vi "Binary_SpectroscopyFile-ExportSlices.vi"() -> ()   [LabVIEW 2016]
doc: "Opens a binary spectroscopy file, then it loops over all spectroscopy experiments doing the following:\n\n - read spectroscopy data\n - extract slices at the specified Sweep signal values in Slices @ control\n - export slices as a scan data file (.sxm, like the files created by the Scan control module) or in\n ASCII format (with a header and several tab-separated data columns)\n\n- Nanonis Programming Interface -"
uses:
  Nanonis Prog Interface.lvlib
  <vilib>/Analysis/NI_AALPro.lvlib
panel:
  in  "Clear Slices array":bool
  in  "Fill Slices array":bool
  out "Points":i32
  out "Sweep signal":string
  out "Sweep End":sgl format="%.2p"
  out "Sweep Start":sgl format="%.2p"
  in  "Export as":enum16{"sxm (scan file)", "ASCII"}(ring)
  out "Status":string
  in  "Filter":bool
  in  "Slices @":dbl[](array[numeric]) caption="m" format="%#_5p"
  in  "Stop":bool
  in  "Channel":u16(ring) items=["Current (A)", "Current [bwd] (A)"]
  in  "Save":bool
  in  "Filter configuration":T1={"Window width\n(# Points for fit)"=20, "Polynomial order"=3}
  out "Error out":errorcluster
  in  "Binary Spectroscopy file path":path
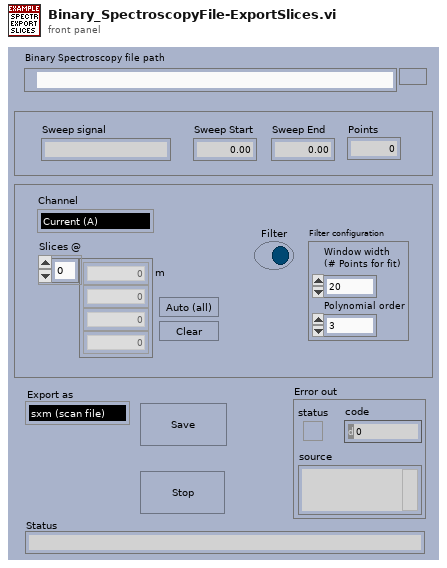
[diagram p1: front panel]
types:
  T1 = cluster{"Window width\n(# Points for fit)":i32, "Polynomial order":i32}
  T2 = enum16{"open", "open or create", "create or replace", "create", "open (read only)"}
  T3 = enum32{"SVD", "Givens", "Givens2", "Householder", "LU Decomposition", "Cholesky"}
  T4 = typedef "Nanonis Prog Interface.lvlib/Binary_SpectroscopyFile-Config.ctl" = cluster{"Num Par":i32, "Exp size":i32, "Points":i32, "Grid Dim X":i32, "Grid Dim Y":i32, "Header size":i32, "Channels":string[], "Parameters":string[], "Sweep Signal":string, "Grid":cluster{"center X (m)":sgl, "center Y (m)":sgl, "width (m)":sgl, "height (m)":sgl, "angle (deg)":sgl}}
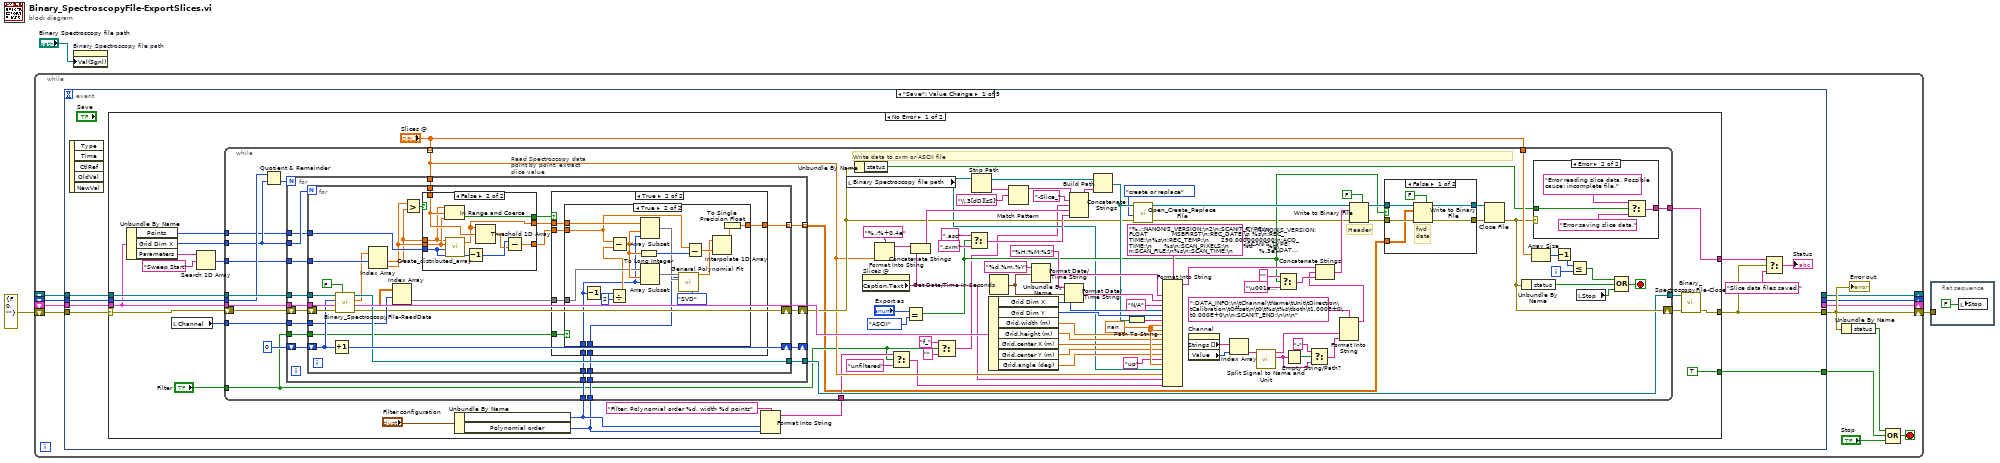
[diagram p0: block diagram]
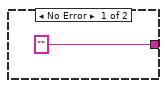
[diagram p2: hidden frame]
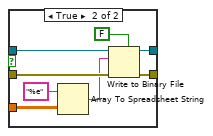
[diagram p3: hidden frame]
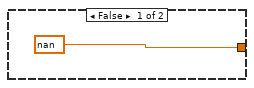
[diagram p4: hidden frame]
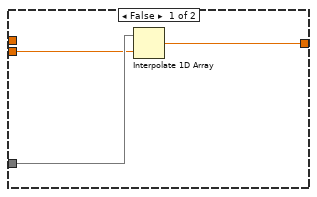
[diagram p5: hidden frame]
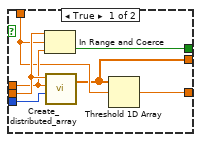
[diagram p6: hidden frame]
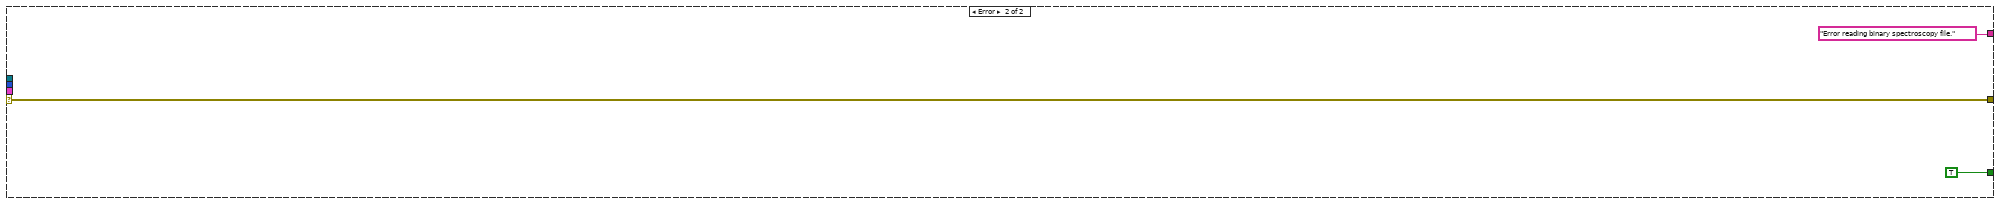
[diagram p7: hidden frame]
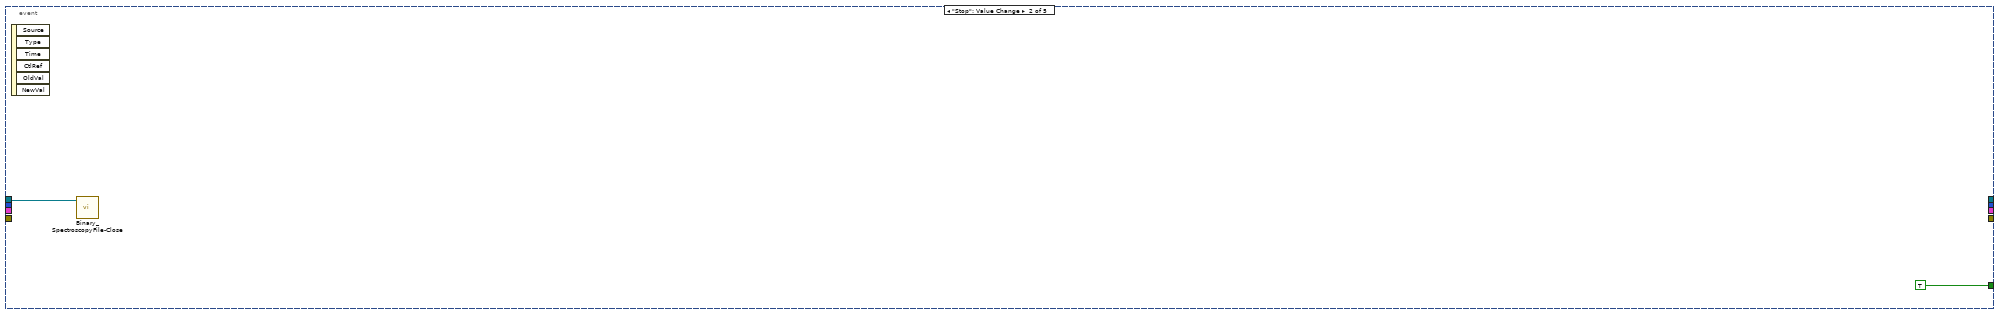
[diagram p8: hidden frame]
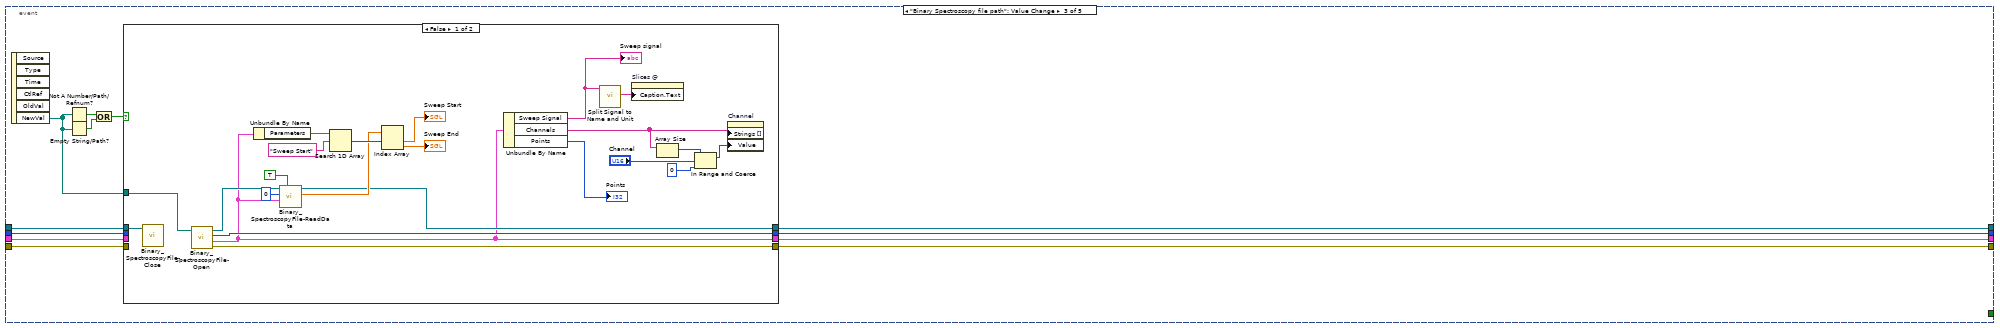
[diagram p9: hidden frame]
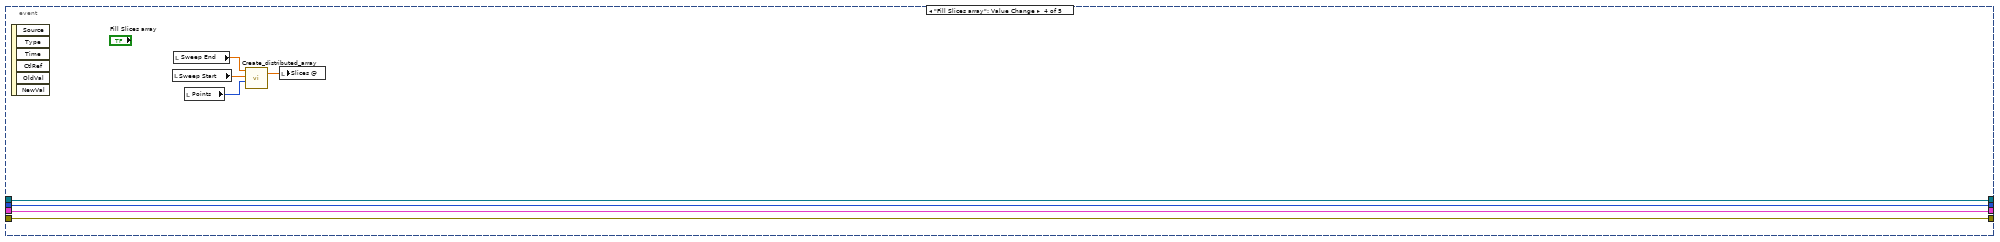
[diagram p11: hidden frame]
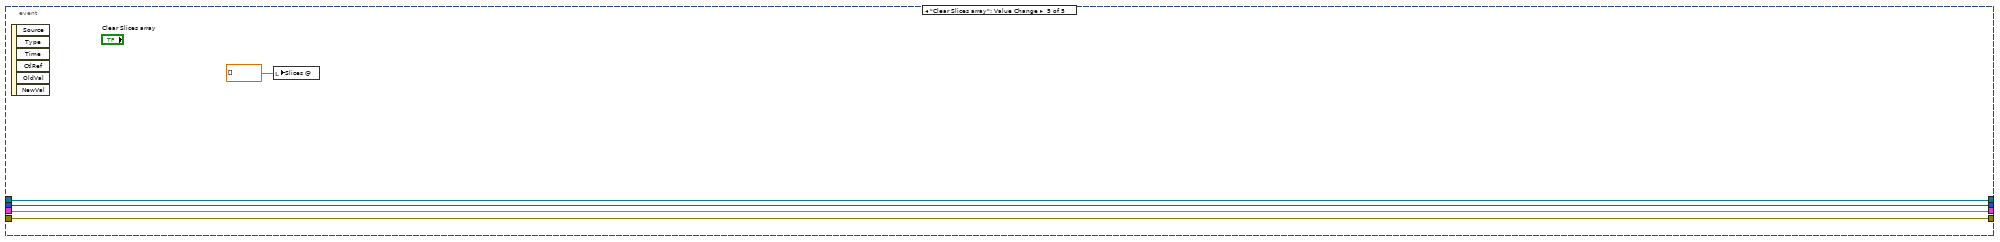
[diagram p12: hidden frame]
diagram:
  n1 = while {
    shift-right: [w4] -> _
    shift-left: _ -> [w8]
    shift-right: [w5] -> _
    shift-left: _ -> [w9]
    shift-right: [w6] -> _
    shift-left: _ -> [w10]
    shift-right: [w7] -> w3
    shift-left: errorcluster {"status"=FALSE, "code"=0, "source"=""} ("error out") -> [w11]
    stop <- w15 stop-if-true
    n2 = event shown="[0] \"Save\": Value Change" {
      selector: _ -> [_ _ _ _ _]
      dyn-events: _ -> [_ _ _ _ _]
      timeout: _ -> [_ _ _ _ _]
      tunnel: [w24 TRUE _ _ _] -> w12
      tunnel: w11 -> [w23 _ w248 w291 w296]
      tunnel: w10 -> [w22 _ w249 w292 w297]
      tunnel: w9 -> [w21 _ w250 w293 w298]
      tunnel: w8 -> [w20 w246 w251 w294 w299]
      tunnel: [w19 _ w256 w291 w296] -> w7
      tunnel: [_ _ w257 w292 w297] -> w6
      tunnel: [_ _ w258 w293 w298] -> w5
      tunnel: [_ _ w259 w294 w299] -> w4
      event "Save": Value Change {
        n3 = event-data() -> ()  [unwired: 1 in, 5 out]
        n4 = case shown="No Error" w23 {
          selector: w23 -> [w31 w243]
          tunnel: w20 -> [w46 _]
          tunnel: w21 -> [w44 _]
          tunnel: w22 -> [w43 _]
          tunnel: [w32 w243] -> w19
          tunnel: [w34 "Error reading binary spectroscopy file." ("Status")] -> w16
          tunnel: [TRUE TRUE] -> w24
          frame No Error {
            n5 = Unbundle By Name(w43) -> ("Points"=w38:i32, "Grid Dim X"=w42:i32, "Parameters"=w40:string[])
            n6 = local read "Channel"() -> (w37:u16)
            n7 = Search 1D Array(1D array=w40, element="Sweep Start" ("string")) -> (index of element=w39:i32)  [unwired: 1 in]
            n8 = Unbundle By Name("Filter configuration") -> ("Window width\n(# Points for fit)"=w28:i32, "Polynomial order"=w27:i32)
            n9 = Format Into String(format string="Filter: Polynomial order %d, width %d points", w28, w27) -> (resulting string=w26:string)  [unwired: 2 in, 1 out]
            n10 = while {
              tunnel: w46 -> [w138]
              tunnel: [w61] -> w45
              tunnel: w44 -> [w136]
              tunnel: w43 -> [w86]
              tunnel: w42 -> [w133]
              tunnel: w39 -> [w132]
              tunnel: "Slices @" -> [w58] mode=indexing
              tunnel: w38 -> [w131]
              tunnel: w37 -> [w130]
              tunnel: w28 -> [w129]
              shift-right: [w63] -> w35
              shift-left: w31 -> [w137]
              tunnel: "Slices @" -> [w127]
              tunnel: [w83] -> w34
              tunnel: w27 -> [w56]
              tunnel: w26 -> [w55]
              tunnel: "Filter" -> [w54]
              i -> [w124]
              stop <- w128 stop-if-true
              w103 = sgl nan ("input 7")
              w87 = "%.;:NANONIS_VERSION:\n2\n:SCANIT_TYPE:\n              FLOAT            MSBFIRST\n:REC_DATE:\n %s\n:REC_TIME:\n%s\n:REC_TEMP:\n      290.0000000000\n:ACQ_TIME:\n      %s\n:SCAN_PIXELS:\n       %d       %d\n:SCAN_FILE:\n%s\n:SCAN_TIME:\n             %.3e             %.3e\n:SCAN_RANGE:\n           %.3e           %.3e\n:SCAN_OFFSET:\n             %.3e         %.3e\n:SCAN_ANGLE:\n            %.3e\n:SCAN_DIR:\n%s\n:BIAS:\n            %.3e\n:COMMENT:\nExported Slice from: %s\nSlice @ %.4e %s\n%s\n"  # %.;:NANONIS_VERSION: 2 :SCANIT_TYPE:               FLOAT            MSBFIRST :REC_DATE:  %s :REC_TIME: %s :REC_TEMP:       290.0000000000 :ACQ_TIME:       %s :SCAN_PIXELS:        %d       %d :SCAN_FILE: %s :SCAN_TIME:              %.3e             %.3e :SCAN_RANGE:            %.3e           %.3e :SCAN_OFFSET:              %.3e         %.3e :SCAN_ANGLE:             %.3e :SCAN_DIR: %s :BIAS:             %.3e :COMMENT: Exported Slice from: %s Slice @ %.4e %s %s
              # "Write data to sxm or ASCII file"
              # "Header"
              n11 = Quotient & Remainder(x=w136, y=w133) -> (floor(x/y)=w135:i32)  [unwired: 1 out]
              n12 = for "Read Spectroscopy data point by point, extract slice value" {
                N: w135 -> [_]
                tunnel: w138 -> [w173]
                tunnel: w86 -> [w171]
                shift-right: [w170] -> w60
                shift-left: w137 -> [w172]
                tunnel: [w169] -> w61
                tunnel: w133 -> [w168]
                shift-right: [w166] -> _
                shift-left: 0 -> [w167]
                tunnel: w132 -> [w165]
                tunnel: w131 -> [w164]
                tunnel: w58 -> [w163]
                tunnel: w130 -> [w162]
                tunnel: [w161] -> w47 mode=indexing
                tunnel: w54 -> [w160]
                tunnel: w129 -> [w159]
                tunnel: w56 -> [w158]
                n13 = for {
                  N: w168 -> [_]
                  tunnel: w173 -> [w198]
                  tunnel: w171 -> [w192]
                  tunnel: [w193] -> w169
                  shift-right: [w178] -> w170
                  shift-left: w172 -> [w197]
                  shift-right: [w194] -> w166
                  shift-left: w167 -> [w195]
                  tunnel: w165 -> [w191]
                  tunnel: w164 -> [w189]
                  tunnel: w163 -> [w188]
                  tunnel: w162 -> [w186]
                  tunnel: [w183] -> w161 mode=indexing
                  tunnel: w160 -> [w181]
                  tunnel: w159 -> [w179]
                  tunnel: w158 -> [w174]
                  n14 = Increment(x=w195) -> (x+1=w194:i32)
                  n15 = call "Binary_SpectroscopyFile-ReadData.vi"("Read Parameters only? (F)"=FALSE, "error in"=w197, "Config"=w192, "Experiment to read (Index)"=w195, "File ref In"=w198) -> ("error out"=w178:errorcluster, "data"=w187:sgl[][], "Parameter values"=w180:sgl[], "File ref Out"=w193:refnum<file>)  [unwired: 3 in]
                  n16 = Index Array(array=w180, index #1=w191) -> (element #1=w176:sgl, element #2=w177:sgl)  [unwired: 1 in]
                  n17 = Index Array(array=w187, index (row)=w186) -> (element=w184:sgl[])  [unwired: 1 in]
                  n18 = Greater?(x=w177, y=w176) -> (0:w190:bool)
                  n19 = case shown="False" w190 {
                    tunnel: [w233 w242] -> w185
                    tunnel: w188 -> [w229 w241]
                    tunnel: w189 -> [w232 w238]
                    tunnel: w177 -> [w231 w240]
                    tunnel: w176 -> [w230 w239]
                    tunnel: [w228 w235] -> w182
                    tunnel: [w227 w234] -> w175
                    frame True {
                      n20 = In Range and Coerce(upper limit=w231, x=w229, lower limit=w230) -> (In Range?=w233:bool)  [unwired: 1 out]
                      n21 = call "Create_distributed_array.vi"("Upper Lim"=w231, "Lower Lim"=w230, "Num Points"=w232) -> ("Array"=w227:dbl[])  [unwired: 3 in]
                      n22 = Threshold 1D Array(2:w229, 3:w227) -> (0:w228:dbl)  [unwired: 1 in]
                    }
                    frame False {
                      n23 = In Range and Coerce(upper limit=w239, x=w241, lower limit=w240) -> (In Range?=w242:bool)  [unwired: 1 out]
                      n24 = call "Create_distributed_array.vi"("Upper Lim"=w239, "Lower Lim"=w240, "Num Points"=w238) -> ("Array"=w234:dbl[])  [unwired: 3 in]
                      n25 = Decrement(x=w238) -> (x-1=w237:i32)
                      n26 = Threshold 1D Array(2:w241, 3:w234) -> (0:w236:dbl)  [unwired: 1 in]
                      n27 = Subtract(x=w237, y=w236) -> (x-y=w235:dbl)
                    }
                  }
                  n28 = case shown="True" w185 {
                    tunnel: w184 -> [_ w206]
                    tunnel: [sgl nan w201] -> w183
                    tunnel: w182 -> [_ w205]
                    tunnel: w181 -> [_ w204]
                    tunnel: w175 -> [_ w203]
                    tunnel: w179 -> [_ w202]
                    tunnel: w174 -> [_ w200]
                    frame False {
                    }
                    frame True {
                      n29 = case shown="True" w204 {
                        tunnel: w206 -> [w209 w224]
                        tunnel: w205 -> [w208 w219]
                        tunnel: w203 -> [_ w225]
                        tunnel: w202 -> [_ w211]
                        tunnel: [w207 w212] -> w201
                        tunnel: w200 -> [_ w210]
                        frame False {
                          n30 = Interpolate 1D Array(1:w208, 2:w209) -> (0:w207:sgl)
                        }
                        frame True {
                          n31 = Decrement(x=w211) -> (x-1=w222:i32)
                          n32 = Divide(x=w222, y=2) -> (x/y=w221:dbl)
                          n33 = Subtract(x=w219, y=w221) -> (x-y=w226:dbl)
                          n34 = To Long Integer(number=w226) -> (32bit integer=w218:i32)
                          n35 = Array Subset(array=w225, index=w226, length=w211) -> (w215:dbl[])
                          n36 = Array Subset(array=w224, index=w226, length=w211) -> (w216:sgl[])
                          n37 = call <vilib>:"General Polynomial Fit.vi"("Y"=w216, "polynomial order"=w210, "X"=w215, "algorithm"=T3."SVD") -> ("Best Polynomial Fit"=w214:dbl[])  [unwired: 8 in, 3 out]
                          n38 = Subtract(x=w219, y=w218) -> (x-y=w220:dbl)
                          n39 = Interpolate 1D Array(1:w220, 2:w214) -> (0:w213:dbl)
                          n40 = To Single Precision Float(number=w213) -> (single precision float=w212:sgl)
                        }
                      }
                    }
                  }
                }
              }
              n41 = local read "Binary Spectroscopy file path"() -> (w51:path)
              n42 = Unbundle By Name(w60) -> ("status"=w82:bool)
              n43 = property on="Slices @" class="Arr (strict)"() -> ("Caption.Text"=w48:string)  [unwired: 2 in, 2 out]
              n44 = Format Into String(format string="%.;%+0.4e", w58) -> (resulting string=w70:string)  [unwired: 2 in, 1 out]
              n45 = Select(t=w55, s=w54, f="unfiltered") -> (s? t:f=w49:string)
              n46 = Equal?(x="Export as", y=enum16{"sxm (scan file)", "ASCII"}."ASCII" ("Export as")) -> (x = y?=w62:bool)
              n47 = Concatenate Strings(w70, w48) -> (w69:string)
              n48 = Select(t="f_", s=w54, f="") -> (s? t:f=w50:string)
              n49 = Select(t=".asc", s=w62, f=".sxm" ("pattern")) -> (s? t:f=w80:string)
              n50 = Strip Path(path=w51) -> (stripped path=w67:path, name=w75:string)
              n51 = Unbundle By Name(w86) -> ("Grid Dim X"=w95:i32, "Grid Dim Y"=w96:i32, "Grid.width (m)"=w97:sgl, "Grid.height (m)"=w98:sgl, "Grid.center X (m)"=w99:sgl, "Grid.center Y (m)"=w100:sgl, "Grid.angle (deg)"=w101:sgl)
              n52 = Get Date/Time In Seconds() -> (seconds since 1Jan1904=w89:timestamp)
              n53 = Match Pattern(string=w75, regular expression="\\.3[dD][sS]") -> (before substring=w76:string)  [unwired: 1 in, 3 out]
              n54 = Format Date/Time String(time format string (%c)="%d.%m.%Y", seconds (now)=w89) -> (date/time string=w92:string)  [unwired: 1 in]
              n55 = Format Date/Time String(time format string (%c)="%H:%M:%S", seconds (now)=w89) -> (date/time string=w93:string)  [unwired: 1 in]
              n56 = Concatenate Strings(w76, "-Slice_" ("string"), w50, w69, w80) -> (w68:string)
              n57 = Build Path(base path=w67, name or relative path=w68) -> (appended path=w66:path)
              n58 = Path To String(path=w66) -> (string=w88:string)
              n59 = call <vilib>:"Open_Create_Replace File.vi"("error in (no error)"=w60, "function (open:0)"=T2."create or replace", "file path"=w66) -> ("error out"=w59:errorcluster, "refnum"=w64:refnum<file>)  [unwired: 5 in, 2 out]
              n60 = Format Into String(format string=w87, w92, w93, "N/A" ("input 3"), w95, w96, w88, w103, w103, w97, w98, w99, w100, w101, "up", w103, w51, w58, w48, w49) -> (resulting string=w113:string)  [unwired: 2 in, 1 out]
              n61 = property on="Channel" class="Ring (strict)"() -> ("Strings []"=w108:string[], "Value"=w107:u16)  [unwired: 2 in, 2 out]
              n62 = Index Array(array=w108, index=w107) -> (element=w110:string)
              n63 = call <userlib>:"Split Signal to Name and Unit.vi"("Name with unit"=w110) -> ("Unit"=w106:string, "Name"=w111:string)  [unwired: 5 in]
              n64 = Select(t="", s=w62, f="\u001a\u0004" ("string")) -> (s? t:f=w121:string)
              n65 = Empty String/Path?(string/path=w106) -> (empty?=w104:bool)
              n66 = Select(t="-", s=w104, f=w106) -> (s? t:f=w112:string)
              n67 = Format Into String(format string=":DATA_INFO:\n\tChannel\tName\tUnit\tDirection\tCalibration\tOffset\n\t0\t%s\t%s\tboth\t1.000E+0\t0.000E+0\n\n:SCANIT_END:\n\n\n", w111, w112) -> (resulting string=w114:string)  [unwired: 2 in, 1 out]
              n68 = Concatenate Strings(w113, w114, w121) -> (w115:string)
              n69 = Write to Binary File(file (use dialog)=w64, data=w115, error in=w59, 5:FALSE ("prepend array or string size? (T)")) -> (refnum out=w116:refnum<file>, error out=w117:errorcluster)  [unwired: 2 in, 1 out]
              n70 = case shown="False" w62 {
                tunnel: w116 -> [w149 w157]
                tunnel: w117 -> [w148 w156]
                tunnel: [w145 w155] -> w118
                tunnel: w47 -> [w147 w153]
                tunnel: [w144 w150] -> w85
                frame False {
                  # "fwd\ndata"
                  n71 = Write to Binary File(file (use dialog)=w149, data=w147, error in=w148, 5:FALSE ("prepend array or string size? (T)")) -> (refnum out=w145:refnum<file>, error out=w144:errorcluster)  [unwired: 2 in, 1 out]
                }
                frame True {
                  n72 = Array To Spreadsheet String(array=w153, 3:"%e" ("format string")) -> (spreadsheet string=w152:string)  [unwired: 1 in]
                  n73 = Write to Binary File(file (use dialog)=w157, data=w152, error in=w156, 5:FALSE ("prepend array or string size? (T)")) -> (refnum out=w155:refnum<file>, error out=w150:errorcluster)  [unwired: 2 in, 1 out]
                }
              }
              n74 = Close File(refnum=w118, error in=w85) -> (error out=w63:errorcluster)  [unwired: 1 out]
              n75 = Unbundle By Name(w63) -> ("status"=w84:bool)
              n76 = Array Size(array=w127) -> (size(s)=w126:i32)
              n77 = case shown="Error" w63 {
                tunnel: ["" ("f") w142] -> w83
                tunnel: w82 -> [_ w141]
                frame No Error {
                }
                frame Error {
                  n78 = Select(t="Error reading slice data. Possible cause: incomplete file." ("Status"), s=w141, f="Error saving slice data." ("Status")) -> (s? t:f=w142:string)
                }
              }
              n79 = Decrement(x=w126) -> (x-1=w125:i32)
              n80 = Less Or Equal?(x=w125, y=w124) -> (x <= y?=w123:bool)
              n81 = local read "Stop"() -> (w81:bool)
              n82 = Compound Arithmetic op=OR(w123, w84, w81) -> (w128:bool)
            }
            n83 = call "Binary_SpectroscopyFile-Close.vi"("error in"=w35, "File ref"=w45) -> ("error out"=w32:errorcluster)  [unwired: 9 in]
          }
          frame Error {
          }
        }
        n84 = Select(t=w16, s=w19, f="Slice data files saved.") -> (s? t:f=→"Status":string)
      }
      event "Stop": Value Change {
        n85 = event-data() -> ()  [unwired: 1 in, 6 out]
        n86 = call "Binary_SpectroscopyFile-Close.vi"("File ref"=w246) -> ()  [unwired: 10 in, 1 out]
      }
      event "Binary Spectroscopy file path": Value Change {
        n87 = event-data() -> ("NewVal"=w255:path)  [unwired: 1 in, 5 out]
        n88 = Not A Number/Path/Refnum?(number/path/refnum=w255) -> (NaN/Path/Refnum?=w254:bool)
        n89 = Empty String/Path?(string/path=w255) -> (empty?=w253:bool)
        n90 = Or(x=w254, y=w253) -> (x .or. y?=w252:bool)
        n91 = case shown="False" w252 {
          tunnel: [w275 w286] -> w259
          tunnel: [w274 w285] -> w258
          tunnel: [w264 w284] -> w257
          tunnel: [w263 w283] -> w256
          tunnel: w255 -> [w261 _]
          tunnel: w251 -> [w260 w286]
          tunnel: w250 -> [_ w285]
          tunnel: w249 -> [_ w284]
          tunnel: w248 -> [_ w283]
          frame False {
            n92 = call "Binary_SpectroscopyFile-Close.vi"("File ref"=w260) -> ()  [unwired: 10 in, 1 out]
            n93 = call "Binary_SpectroscopyFile-Open.vi"("Binary Spectroscopy File"=w261) -> ("error out"=w263:errorcluster, "Config"=w264:T4, "Number of Experiments"=w274:i32, "File ref"=w282:refnum<file>)  [unwired: 6 in, 1 out]
            n94 = Unbundle By Name(w264) -> ("Parameters"=w279:string[])
            n95 = call "Binary_SpectroscopyFile-ReadData.vi"("Read Parameters only? (F)"=TRUE, "Config"=w264, "Experiment to read (Index)"=0, "File ref In"=w282) -> ("Parameter values"=w280:sgl[], "File ref Out"=w275:refnum<file>)  [unwired: 4 in, 2 out]
            n96 = Search 1D Array(1D array=w279, element="Sweep Start" ("string")) -> (index of element=w281:i32)  [unwired: 1 in]
            n97 = Index Array(array=w280, index #1=w281) -> (element #1=→"Sweep Start":sgl, element #2=→"Sweep End":sgl)  [unwired: 1 in]
            n98 = Unbundle By Name(w264) -> ("Sweep Signal"=w267:string, "Channels"=w271:string[], "Points"=→"Points":i32)
            "Sweep signal" <- w267
            n99 = call <userlib>:"Split Signal to Name and Unit.vi"("Name with unit"=w267) -> ("Unit"=w268:string)  [unwired: 5 in, 1 out]
            n100 = property on="Slices @" class="Arr (strict)"("Caption.Text"=w268) -> ()  [unwired: 2 in, 2 out]
            n101 = Array Size(array=w271) -> (size(s)=w272:i32)
            n102 = In Range and Coerce(upper limit=w272, x="Channel", lower limit=0) -> (coerced(x)=w270:i32)  [unwired: 1 out]
            n103 = property on="Channel" class="Ring (strict)"("Strings []"=w271, "Value"=w270) -> ()  [unwired: 2 in, 2 out]
          }
          frame True {
          }
        }
      }
      event "Fill Slices array": Value Change {
        n104 = event-data() -> ()  [unwired: 1 in, 6 out]
        n105 = local read "Sweep Start"() -> (w289:sgl)
        n106 = local read "Sweep End"() -> (w290:sgl)
        n107 = local read "Points"() -> (w288:i32)
        n108 = call "Create_distributed_array.vi"("Upper Lim"=w290, "Lower Lim"=w289, "Num Points"=w288) -> ("Array"=w287:dbl[])  [unwired: 3 in]
        n109 = local write "Slices @"(w287) -> ()
      }
      event "Clear Slices array": Value Change {
        n110 = event-data() -> ()  [unwired: 1 in, 6 out]
        n111 = local write "Slices @"(dbl[] [] ("Slices @")) -> ()
      }
    }
    "Error out" <- w7
    n112 = Unbundle By Name(w7) -> ("status"=w14:bool)
    n113 = Compound Arithmetic op=OR(w14, w12, "Stop") -> (w15:bool)
  }
  n114 = property on="Binary Spectroscopy file path" class="Path"("Val(Sgnl)"="Binary Spectroscopy file path") -> ()  [unwired: 2 in, 2 out]
  n115 = flat-sequence {
    tunnel: w3 -> [_]
    frame #0 {
      n116 = local write "Stop"(FALSE ("Stop")) -> ()
    }
  }
